vi "temp_subvi_position.vi"(0 "Position Reset":bool, 1 "Length of the FCM (m)":dbl, 2 "Radius of disk (m)":dbl, 3 "Number of Disks":dbl, 4 "Tip position":dbl[](array[numeric]), 7 "Radius of pulley (mm)":dbl) -> (8 "L1 (m)":dbl, 9 "alpha":dbl, 10 "output variable":dbl, 11 "L_v":dbl, 12 "L2 (m)":dbl, 13 "Theta 3":dbl, 14 "output variable 2":dbl, 15 "Theta 1":dbl, 16 "Theta 2":dbl, 17 "L3 (m)":dbl, 18 "output variable 3":dbl)   [LabVIEW 2019]
uses:
  <vilib>/FPGAPlugInAG/sbRIO-9629/niLvFpga_Open_sbRIO-9629.vi
  <vilib>/rvi/interface/common/dynamic/niFpgaDynamicAddResources.vi
  <vilib>/imath/engines/lvmath2/RunTimeEngine/Managers/WorkSpace/UID Generator.vi
  <vilib>/imath/engines/lvmath2/RunTimeEngine/RunTimeType/NIMS_RunTimeType_From StrictType (excl LVString).vi
  <instcachedir>/0/NIMS_RunTimeType_From StrictType (excl LVString)_D8AFBA86A94845AAA577C895450664BD.lvgen/NIMS_RunTimeType_From StrictType (excl LVString)_D8AFBA86A94845AAA577C895450664BD_000.vi
  <vilib>/imath/engines/lvmath2/RunTimeEngine/LocalVariableDefStatement/MC_LocalVariableDefStatement_Display.vi
  <vilib>/imath/engines/lvmath2/RunTimeEngine/IndexRead/NIMS V(S).vi
  <instcachedir>/0/NIMS V(S)_0488751826AF41519A22953C041130DC.lvgen/NIMS V(S)_0488751826AF41519A22953C041130DC_000.vi
  <vilib>/imath/engines/lvmath2/RunTimeEngine/BuiltInFunctions/atan2/NIMS_atan2.vi
  <instcachedir>/0/NIMS_atan2_A91AA4A7D42247EDBE8F76DB99AF04A4.lvgen/NIMS_atan2_A91AA4A7D42247EDBE8F76DB99AF04A4_000.vi
  <vilib>/imath/engines/lvmath2/RunTimeEngine/ErrorHandling/NIMS_Create Error From Enums.vi
  <vilib>/imath/engines/lvmath2/RunTimeEngine/BuiltInFunctions/atan/NIMS_atan(C).vi
  <instcachedir>/0/NIMS_atan(C)_0A85D365582D4E8AB3874BC9125E138E.lvgen/NIMS_atan(C)_0A85D365582D4E8AB3874BC9125E138E_001.vi
  <vilib>/imath/engines/lvmath2/RunTimeEngine/BuiltInFunctions/cross/NIMS_cross(GV,GV).vi
  <instcachedir>/0/NIMS_cross(GV,GV)_6F1F1C643EFF41C8A983D972A94A5A15.lvgen/NIMS_cross(GV,GV)_6F1F1C643EFF41C8A983D972A94A5A15_000.vi
  <vilib>/imath/engines/lvmath2/RunTimeEngine/BuiltInFunctions/norm/NIMS_norm(GV,DBL).vi
  <instcachedir>/0/NIMS_norm(GV,DBL)_4A8B6F23BC0A47549B8AB805006257D9.lvgen/NIMS_norm(GV,DBL)_4A8B6F23BC0A47549B8AB805006257D9_000.vi
  <vilib>/imath/engines/lvmath2/RunTimeEngine/ArithmeticOperatorToken/NIMS_ArithmeticOperator_multmx-internal.vi
  <instcachedir>/0/NIMS_ArithmeticOperator_multmx-internal_9E91BA3A2DCB4083AAD724A04442A6F7.lvgen/NIMS_ArithmeticOperator_multmx-internal_9E91BA3A2DCB4083AAD724A04442A6F7_004.vi
  <vilib>/imath/engines/lvmath2/RunTimeEngine/BuiltInFunctions/cos/NIMS_cos(C).vi
  <instcachedir>/0/NIMS_cos(C)_BED070B05FDB4939A63CB05E18805866.lvgen/NIMS_cos(C)_BED070B05FDB4939A63CB05E18805866_001.vi
  <vilib>/imath/engines/lvmath2/RunTimeEngine/BuiltInFunctions/sin/NIMS_sin(C).vi
  <instcachedir>/0/NIMS_sin(C)_6504C6AC704B4661870B0E93397B11C4.lvgen/NIMS_sin(C)_6504C6AC704B4661870B0E93397B11C4_001.vi
  <vilib>/imathl/engines/lvmath/Functions/Error Handling/Create Error.vi
  <vilib>/imath/engines/lvmath2/RunTimeEngine/ArithmeticOperatorToken/NIMS_ArithmeticOperator_multmx(M,CV)-internal.vi
  <instcachedir>/0/NIMS_ArithmeticOperator_multmx(M,CV)-internal_2C55777844884EEDB828A940D397C7D0.lvgen/NIMS_ArithmeticOperator_multmx(M,CV)-internal_2C55777844884EEDB828A940D397C7D0_002.vi
  <instcachedir>/0/NIMS_norm(GV,DBL)_4A8B6F23BC0A47549B8AB805006257D9.lvgen/NIMS_norm(GV,DBL)_4A8B6F23BC0A47549B8AB805006257D9_001.vi
  <vilib>/imath/engines/lvmath2/RunTimeEngine/Managers/SymbolTable/Clear UID.vi
  <vilib>/imath/engines/lvmath2/RunTimeEngine/NodeEndStatement/NIMS_NodeEndStatement_Output.vi
  <instcachedir>/0/NIMS_NodeEndStatement_Output_53EC0D466D134D7ABD903AC30B43404B.lvgen/NIMS_NodeEndStatement_Output_53EC0D466D134D7ABD903AC30B43404B_001.vi
  <vilib>/imath/engines/lvmath2/RunTimeEngine/ErrorHandling/NIMS_Finalize Error.vi
  <vilib>/Utility/error.llb/Error Cluster From Error Code.vi
  <vilib>/rvi/errors/niLvFpgaAdjustHostInterfaceError.vi
  <vilib>/FPGAPlugInAG/Dynamic/niLvFpga_Close_Dynamic.vi
  <vilib>/rvi/interface/nirviOpenFPGA/nirviOpenFPGA.xnode
  FPGA Bitfiles/fcmsinglesection_FPGATarget_CloseLoopMotorTu_eGt+d+EV+VE.lvbitx
  Close_Loop_Motor_Tune.vi
  <vilib>/rvi/interface/nirviReadWriteControl/nirviReadWriteControl.xnode
  <vilib>/rvi/interface/nirviCloseFPGA/nirviCloseFPGA.xnode
  NiFpgaLv.dll
  <vilib>/rvi/interface/Simulation/niFpgaSimulationCallBeginRW.vi
  <vilib>/imath/engines/lvmath2/RunTimeEngine/Managers/SymbolTable/NIMS_WorkSpace.lvlib
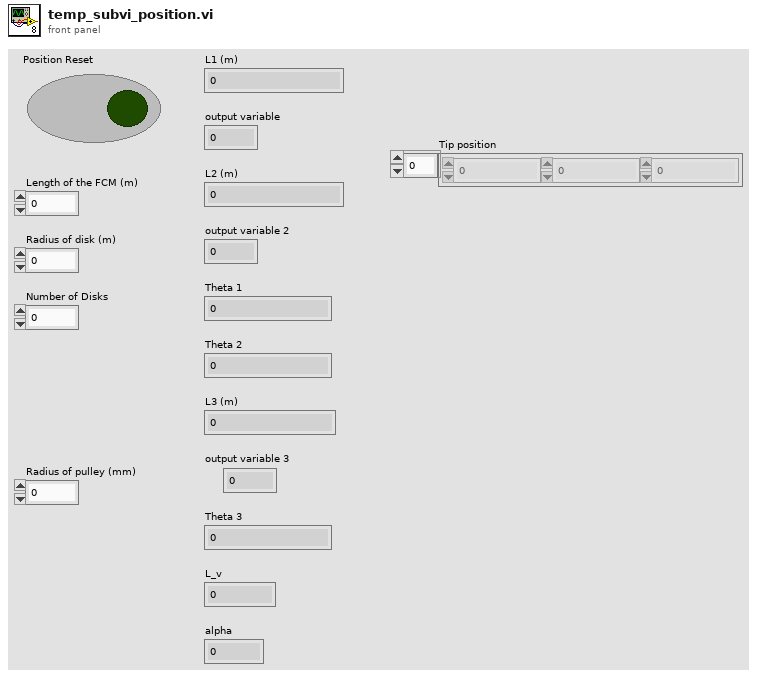
[diagram p1: front panel]
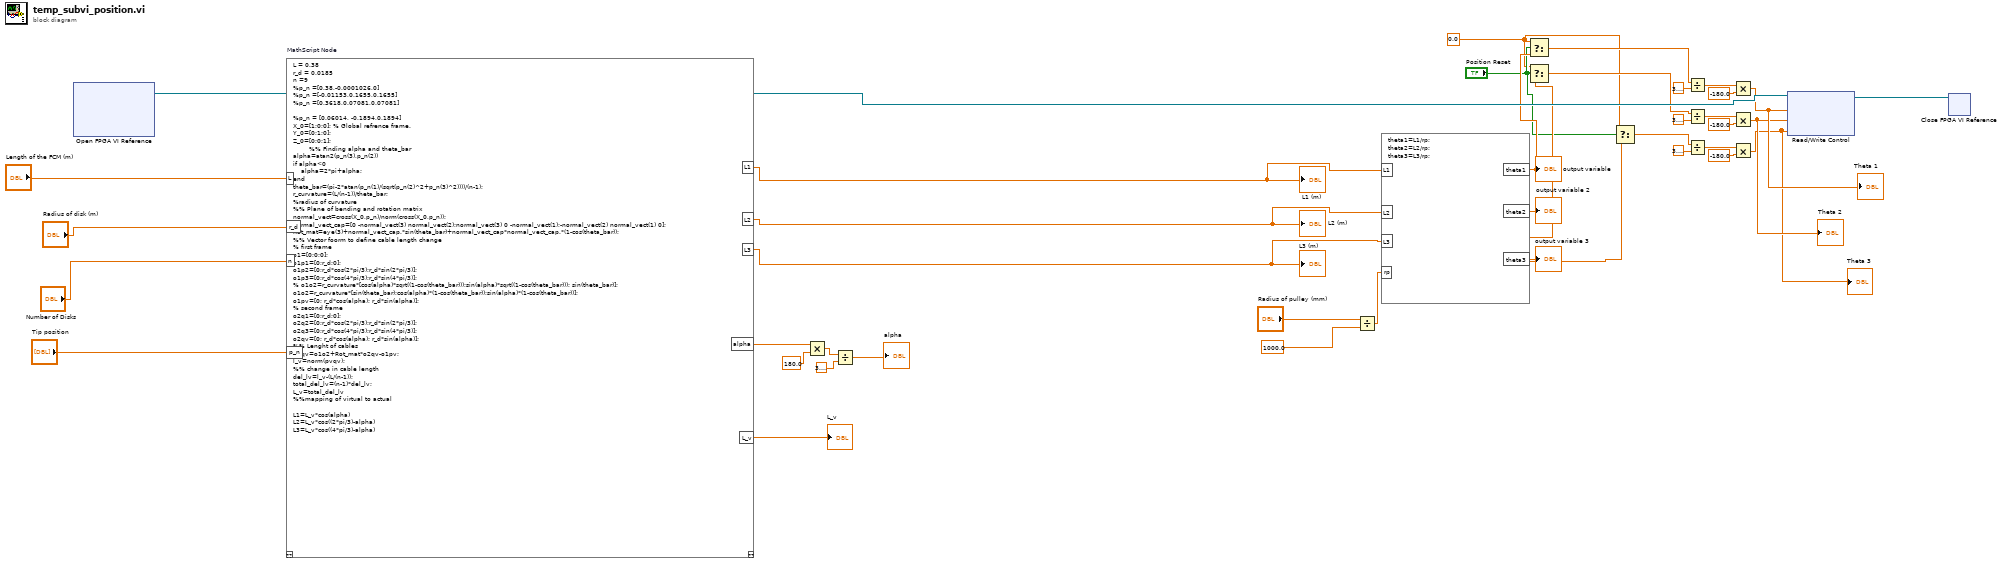
[diagram p0: block diagram]
diagram:
  w13 = 0.0 ("t")
  n1 = xnode "Open FPGA VI Reference"() -> ("FPGA VI Reference Out"=w33:refnum<k20>)  [unwired: 2 in, 1 out]
  n2 = mathscript code="L = 0.38\nr_d = 0.0185\nn =9\n%p_n =[0.38,-0.0001026,0] \n%p_n =[-0.01153,0.1655,0.1655] \n%p_n =[0.3618,0.07081,0.07081] \n\n%p_n = [0.06014, -0.1894,0.1894]\nX_0=[1;0;0]; % Global refrence frame.\nY_0=[0;1;0];\nZ_0=[0;0;1];\n        %% Finding alpha and theta_bar\nalpha=atan2(p_n(3),p_n(2))\nif alpha<0\n    alpha=2*pi+alpha;\nend\ntheta_bar=(pi-2*atan(p_n(1)/(sqrt(p_n(2)^2+p_n(3)^2))))/(n-1);\nr_curvature=(L/(n-1))/theta_bar; \n%radius of curvature\n%% Plane of bending and rotation matrix\nnormal_vect=cross(X_0,p_n)/norm(cross(X_0,p_n));\nnormal_vect_cap=[0 -normal_vect(3) normal_vect(2);normal_vect(3) 0 -normal_vect(1);-normal_vect(2) normal_vect(1) 0];\nRot_mat=eye(3)+normal_vect_cap.*sin(theta_bar)+normal_vect_cap*normal_vect_cap.*(1-cos(theta_bar));\n%% Vector foorm to define cable length change\n% first frame\no1=[0;0;0];\no1p1=[0;r_d;0];\no1p2=[0;r_d*cos(2*pi/3);r_d*sin(2*pi/3)];\no1p3=[0;r_d*cos(4*pi/3);r_d*sin(4*pi/3)];\n% o1o2=r_curvature*[cos(alpha)*sqrt((1-cos(theta_bar)));sin(alpha)*sqrt((1-cos(theta_bar))); sin(theta_bar)];\no1o2=r_curvature*[sin(theta_bar);cos(alpha)*(1-cos(theta_bar));sin(alpha)*(1-cos(theta_bar))];\no1pv=[0; r_d*cos(alpha); r_d*sin(alpha)];\n% second frame\no2q1=[0;r_d;0];\no2q2=[0;r_d*cos(2*pi/3);r_d*sin(2*pi/3)];\no2q3=[0;r_d*cos(4*pi/3);r_d*sin(4*pi/3)];\no2qv=[0; r_d*cos(alpha); r_d*sin(alpha)];\n%% Lenght of cables\npvqv=o1o2+Rot_mat*o2qv-o1pv;\nl_v=norm(pvqv);\n%% change in cable length\ndel_lv=l_v-(L/(n-1));\ntotal_del_lv=(n-1)*del_lv;\nL_v=total_del_lv\n%%mapping of virtual to actual\n\nL1=L_v*cos(alpha)\nL2=L_v*cos((2*pi/3)-alpha)\nL3=L_v*cos((4*pi/3)-alpha)"("L"="Length of the FCM (m)", "r_d"="Radius of disk (m)", "n"="Number of Disks", "p_n"="Tip position") -> ("L_v"=→"L_v":dbl, "alpha"=w6:dbl, "L1"=w3:dbl, "L2"=w2:dbl, "L3"=w1:dbl)  [unwired: 1 in, 1 out]
  "L1 (m)" <- w3
  "L2 (m)" <- w2
  "L3 (m)" <- w1
  n3 = Multiply(x=w6, y=180.0) -> (x*y=w8:dbl)
  n4 = Divide(x=w8, y=3.141592653589793) -> (x/y=→"alpha":dbl)
  n5 = Divide(x="Radius of pulley (mm)", y=1000.0) -> (x/y=w32:dbl)
  n6 = formula code="theta1=L1/rp;\ntheta2=L2/rp;\ntheta3=L3/rp;"("L1"=w3, "L2"=w2, "L3"=w1, "rp"=w32) -> ("theta1"=w20:dbl, "theta2"=w17:dbl, "theta3"=w15:dbl)
  "output variable" <- w20
  "output variable 2" <- w17
  "output variable 3" <- w15
  n7 = Select(t=w13, s="Position Reset", f=w20) -> (s? t:f=w19:dbl)
  n8 = Select(t=w13, s="Position Reset", f=w17) -> (s? t:f=w18:dbl)
  n9 = Select(t=w13, s="Position Reset", f=w15) -> (s? t:f=w16:dbl)
  n10 = Divide(x=w19, y=3.141592653589793) -> (x/y=w28:dbl)
  n11 = Divide(x=w18, y=3.141592653589793) -> (x/y=w25:dbl)
  n12 = Divide(x=w16, y=3.141592653589793) -> (x/y=w22:dbl)
  n13 = Multiply(x=w28, y=-180.0) -> (x*y=w12:dbl)
  "Theta 1" <- w12
  n14 = Multiply(x=w25, y=-180.0) -> (x*y=w11:dbl)
  "Theta 2" <- w11
  n15 = Multiply(x=w22, y=-180.0) -> (x*y=w10:dbl)
  "Theta 3" <- w10
  n16 = xnode "Read/Write Control"("FPGA VI Reference In"=w33, "desired angle"=w12, "desired angle 2"=w11, "desired angle 3"=w10) -> ("FPGA VI Reference Out"=w34:refnum<k20>)  [unwired: 1 in, 1 out]
  n17 = xnode "Close FPGA VI Reference"("FPGA VI Reference In"=w34) -> ()  [unwired: 1 in, 1 out]
